vi "send_reply.vi"(8 "error in (no error)":errorcluster, 10 "message":T1, 11 "client in":refnum<class "client.lvclass">) -> (0 "error out":errorcluster, 3 "client out":refnum<class "client.lvclass">)   [LabVIEW 2020, in "client.lvclass"]
uses:
  client.lvclass
  shared/message--cluster.ctl
  shared/request--enum.ctl
  client.lvclass/client.ctl
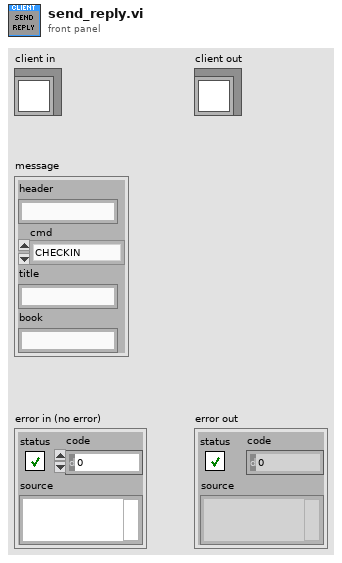
[diagram p1: front panel]
types:
  T1 = typedef "message--cluster.ctl" = cluster{"header":string, "cmd":T2, "title":string, "book":string}
  T2 = typedef "request--enum.ctl" = enum16{"CHECKIN", "CHECKOUT"}
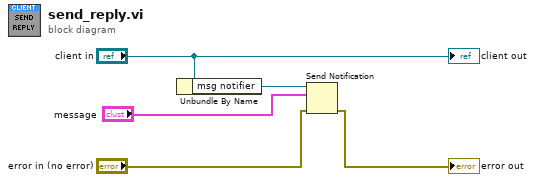
[diagram p0: block diagram]
diagram:
  n1 = Unbundle By Name("client in") -> ("msg notifier"=w4:refnum<notifier>)
  n2 = Send Notification(notification="message", notifier=w4, error in (no error)="error in (no error)") -> (error out=→"error out":errorcluster)  [unwired: 1 out]
  "client out" <- "client in"
